vi "create image name.vi"(8 "error in (no error)":errorcluster, 11 "Channel in":refnum<class "Channel.lvclass">) -> (0 "error out":errorcluster, 3 "Channel out":refnum<class "Channel.lvclass">)   [LabVIEW 2018, in "Channel.lvclass"]
uses:
  Channel.lvclass
  Channel.lvclass/Channel.ctl
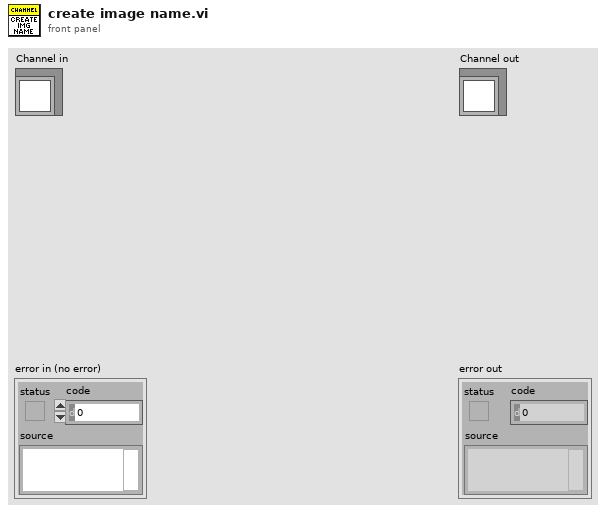
[diagram p1: front panel]
types:
  T1 = typedef "LVDateTimeRec.ctl" = cluster{"fractional second":dbl, "second":i32, "minute":i32, "hour":i32, "day of month":i32, "month":i32, "year":i32, "day of week":i32, "day of year":i32, "DST":i32}
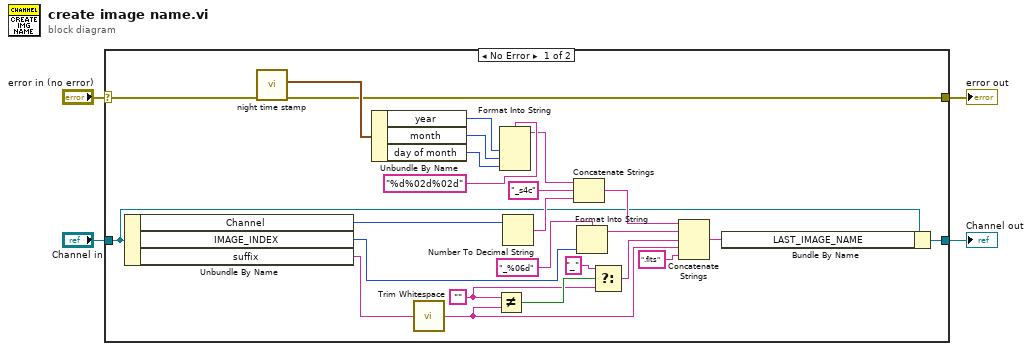
[diagram p0: block diagram]
diagram:
  n1 = case shown="No Error" "error in (no error)" {
    selector: "error in (no error)" -> [w10 w31]
    tunnel: [w9 w31] -> w3
    tunnel: [w7 w30] -> w1
    tunnel: "Channel in" -> [w8 w30]
    frame No Error {
      w20 = ""
      n2 = Unbundle By Name(w8) -> ("Channel"=w5:u8, "IMAGE_INDEX"=w12:u32, "suffix"=w6:string)
      n3 = call "night time stamp.vi"("error in (no error)"=w10) -> ("error out"=w9:errorcluster, "date time rec"=w11:T1)  [unwired: 9 in]
      n4 = Unbundle By Name(w11) -> ("year"=w19:i32, "month"=w18:i32, "day of month"=w13:i32)
      n5 = call <vilib>:"Trim Whitespace.vi"("string"=w6) -> ("trimmed string"=w16:string)  [unwired: 1 in]
      n6 = Not Equal?(x=w20, y=w16) -> (x != y?=w26:bool)
      n7 = Format Into String(format string="%d%02d%02d", w19, w18, w13) -> (resulting string=w21:string)  [unwired: 2 in, 1 out]
      n8 = Number To Decimal String(number=w5) -> (decimal integer string=w28:string)  [unwired: 1 in]
      n9 = Concatenate Strings(w21, "_s4c" ("string"), w28) -> (w27:string)
      n10 = Format Into String(format string="_%06d", w12) -> (resulting string=w15:string)  [unwired: 2 in, 1 out]
      n11 = Select(t="_" ("string"), s=w26, f=w20) -> (s? t:f=w14:string)
      n12 = Concatenate Strings(w27, w15, w14, w16, ".fits" ("string")) -> (w17:string)
      n13 = Bundle By Name(cluster=w8, "LAST_IMAGE_NAME"=w17) -> (w7:refnum<class "Channel.lvclass">)
    }
    frame Error {
    }
  }
  "error out" <- w3
  "Channel out" <- w1
